vi "Initialize Galil 2.vi"(0 "Galil.IGalil":refnum<k7>, 1 "Command Input":string="0" caption="Enter number in encoder counts, 0 is middle, -650000 fully entended; 650000 fully retracted", 12 "Disabled?":bool) -> (4 "reference out 3":refnum<k7>, 5 "address":string="192.168.1.10", 6 "error out 3":errorcluster, 9 "timeout_ms":i32=500, 14 "Output String":string, 15 "Error Query Connection":errorcluster)   [LabVIEW 2011]
panel:
  out "error out 2":errorcluster
  out "addresses":variant
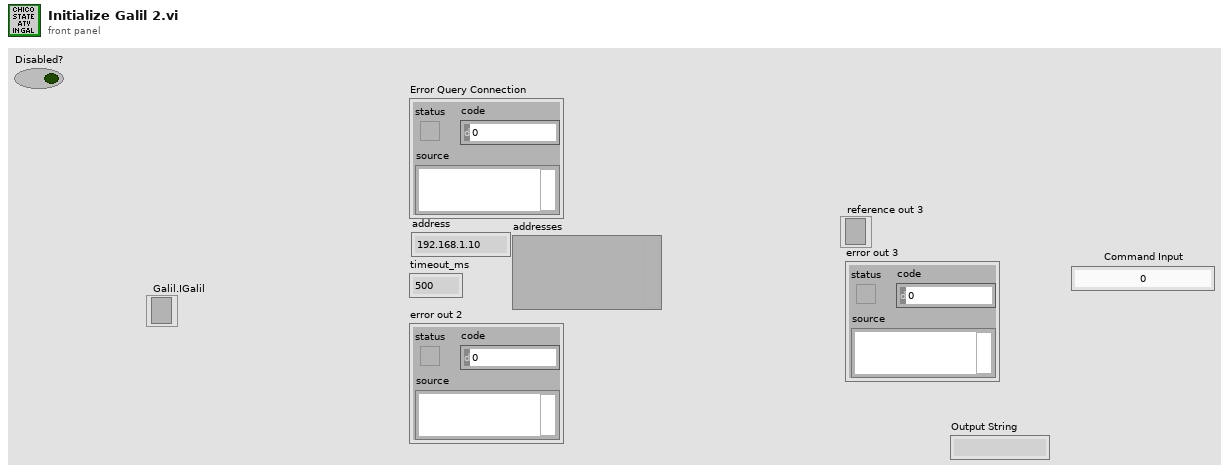
[diagram p1: front panel]
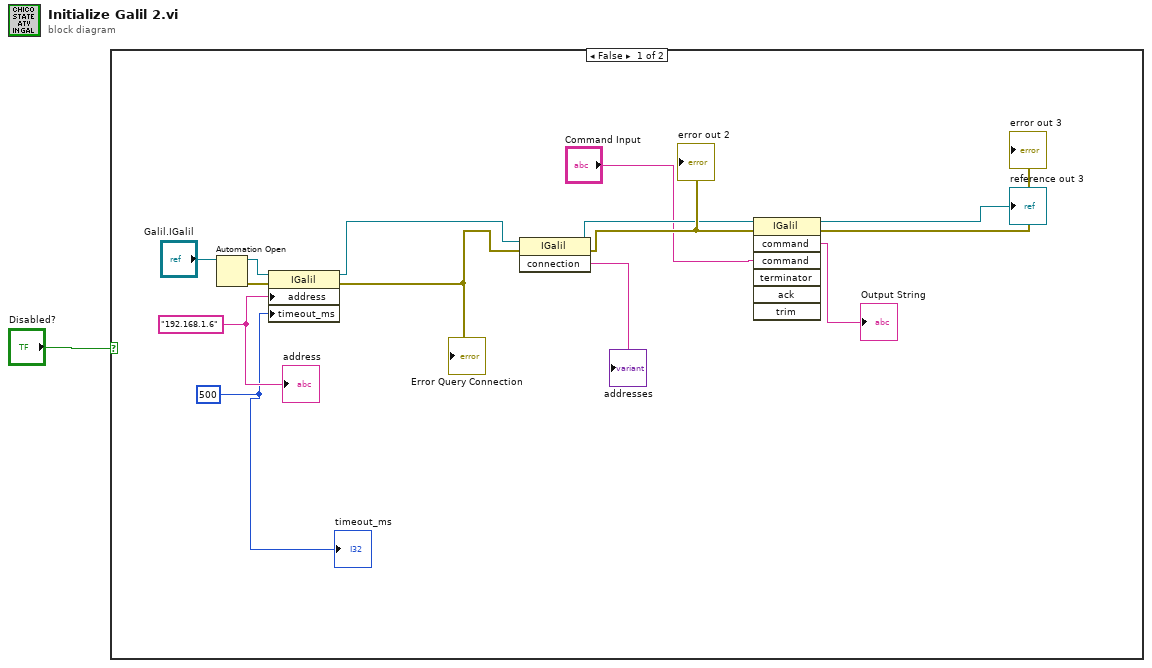
[diagram p0: block diagram]
diagram:
  n1 = case shown="False" "Disabled?" {
    frame False {
      w3 = 500 ("timeout_ms")
      w4 = "192.168.1.6" ("address")
      n2 = Automation Open(Automation Refnum="Galil.IGalil") -> (Automation Refnum=w12:refnum<k7>, error out=w11:errorcluster)  [unwired: 3 in]
      n3 = property class="IGalil"(reference=w12, error in=w11, "address"=w4, "timeout_ms"=w3) -> (reference out=w8:refnum<k7>, error out=w9:errorcluster)
      "Error Query Connection" <- w9
      n4 = invoke class="IGalil" method="connection"(reference=w8, error in=w9) -> (reference out=w5:refnum<k7>, error out=w6:errorcluster, "connection"=→"addresses":string)  [unwired: 1 in]
      "error out 2" <- w6
      n5 = invoke class="IGalil" method="command"(reference=w5, error in=w6, "command"="Command Input") -> (reference out=→"reference out 3":refnum<k7>, error out=→"error out 3":errorcluster, "command"=→"Output String":string)  [unwired: 4 in, 4 out]
      "address" <- w4
      "timeout_ms" <- w3
    }
    frame True {
    }
  }
